vi "WriteU64ToU16FIFO.vi"(1 "U64":u64) -> ()   [LabVIEW 2018]
uses:
  <vilib>/rvi/interface/RandomDataEmulation/niFpgaRandomDataHandleErrors.vi
  <vilib>/rvi/DataTransferAndStorage/Container/Common/niFpgaContainerExecOnDevCompGetState.vi
  <vilib>/rvi/Emulation/niFpgaEmulationIsFPGAContextNoSignature.vi
  <vilib>/rvi/Emulation/niFpgaSctlEmulationGetInTimedLoop.vi
  <vilib>/rvi/errors/niFpgaSetErrorForExecOnDevCompSimple.vi
  <vilib>/rvi/eio/common/nirviEmuReportErrorAndStop.vi
  <vilib>/rvi/DataTransferAndStorage/Container/Common/niFpgaContainerGetUniqueNameForEmu.vi
  <vilib>/rvi/FIFO/Fifo_Resource/nirvififoEmulationSetSize.vi
  <vilib>/rvi/FIFO/Fifo_Resource/nirviFifoEmulationQueueMgr.vi
  <instcachedir>/0/nirviFifoEmulationQueueMgr_E5CAEC123FF24DC58D834DCA3CDAA9B5.lvgen/nirviFifoEmulationQueueMgr_E5CAEC123FF24DC58D834DCA3CDAA9B5_012.vi
  <vilib>/rvi/FIFO/Fifo_Resource/nirvififoEmulationDetermineInputValidOut.vi
  <vilib>/rvi/FIFO/Fifo_Resource/nirvififoEmulationCreateLock.vi
  <vilib>/rvi/Emulation/niFpgaProcessEmulError.vi
  <vilib>/rvi/FIFO/Fifo_Resource/nirvififoEmulationObtainLock.vi
  <vilib>/rvi/FIFO/Fifo_Resource/nirvififoEmulationReleaseLock.vi
  <vilib>/rvi/occurrence/nirviWaitOnOccurrenceBase.vi
  <vilib>/rvi/errors/nirviReportUnexpectedCaseInternalError.vi
  <vilib>/rvi/errors/nirviReportUnexpectedCaseInternalError (U32).vi
  <vilib>/Utility/error.llb/Clear Errors.vi
  <vilib>/rvi/DataTransferAndStorage/Container/XNode/niFpgaContainer.xnode
  <vilib>/rvi/interface/RandomDataEmulation/nirviRandomDataFpgaReadWriteTemplate.vi
  <vilib>/rvi/FIFO/Fifo_Resource/niFpgaFifoEmulationRefIn.vi
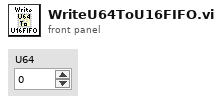
[diagram p1: front panel]
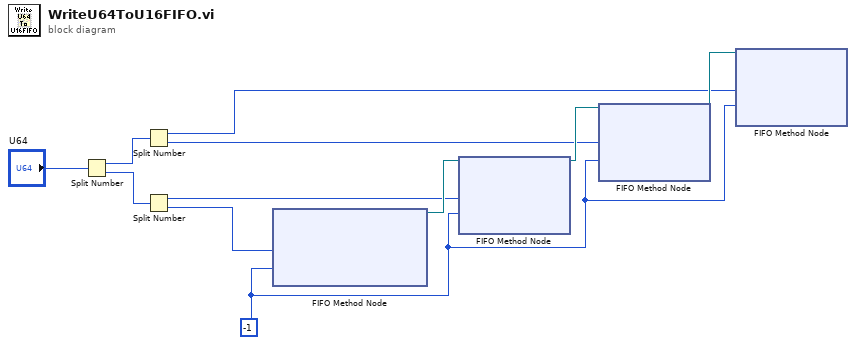
[diagram p0: block diagram]
diagram:
  w5 = -1 ("Timeout")
  n1 = Split Number(x="U64") -> (hi(x)=w6:u32, lo(x)=w7:u32)
  n2 = Split Number(x=w6) -> (hi(x)=w4:u16, lo(x)=w3:u16)
  n3 = Split Number(x=w7) -> (hi(x)=w2:u16, lo(x)=w1:u16)
  n4 = xnode ("FIFO Method Node")("Element"=w1, "Timeout"=w5) -> ("FIFO Out"=w11:refnum<k21>)  [unwired: 1 in, 1 out]
  n5 = xnode ("FIFO Method Node")("Element"=w2, "Timeout"=w5, "FIFO In"=w11) -> ("FIFO Out"=w10:refnum<k21>)  [unwired: 1 out]
  n6 = xnode ("FIFO Method Node")("Element"=w3, "Timeout"=w5, "FIFO In"=w10) -> ("FIFO Out"=w9:refnum<k21>)  [unwired: 1 out]
  n7 = xnode ("FIFO Method Node")("Element"=w4, "Timeout"=w5, "FIFO In"=w9) -> ()  [unwired: 2 out]
